vi "Post Media Tweet - From File.vi"(8 "error in":errorcluster, 9 "Picture File (PNG, JPG, GIF)":path, 10 "Tweet":string, 11 "Twitter Handle In":T1={"OAuth Credentials"={"Consumer Key"="", "Signature Method"=enum."HMAC-SHA1", "Token"="", "Version"="", "Token Secret"="", "Consumer Secret"=""}, "since ID"="", "max ID"="", "Screen Name"=""}) -> (0 "error out":errorcluster, 3 "Twitter Handle Out":T1={"OAuth Credentials"={"Consumer Key"="", "Signature Method"=enum."HMAC-SHA1", "Token"="", "Version"="", "Token Secret"="", "Consumer Secret"=""}, "since ID"="", "max ID"="", "Screen Name"=""})   [LabVIEW 2011, in "i3-twitter.lvlib"]
uses:
  i3-twitter.lvlib
  Controls/Twitter Handle.ctl
  i3-oauth/Controls/OAuth Credentials.ctl
  i3-oauth/Controls/Signature Method.ctl
  <vilib>/httpClient/MultipartData.ctl
  i3-oauth/Controls/HTTP Method.ctl
  i3-oauth/i3-oauth.lvlib
  <vilib>/httpClient/LabVIEWHTTPClient.lvlib
panel:
  out "headers (response)":string
  out "body (response)":string
  out "Full URL":string
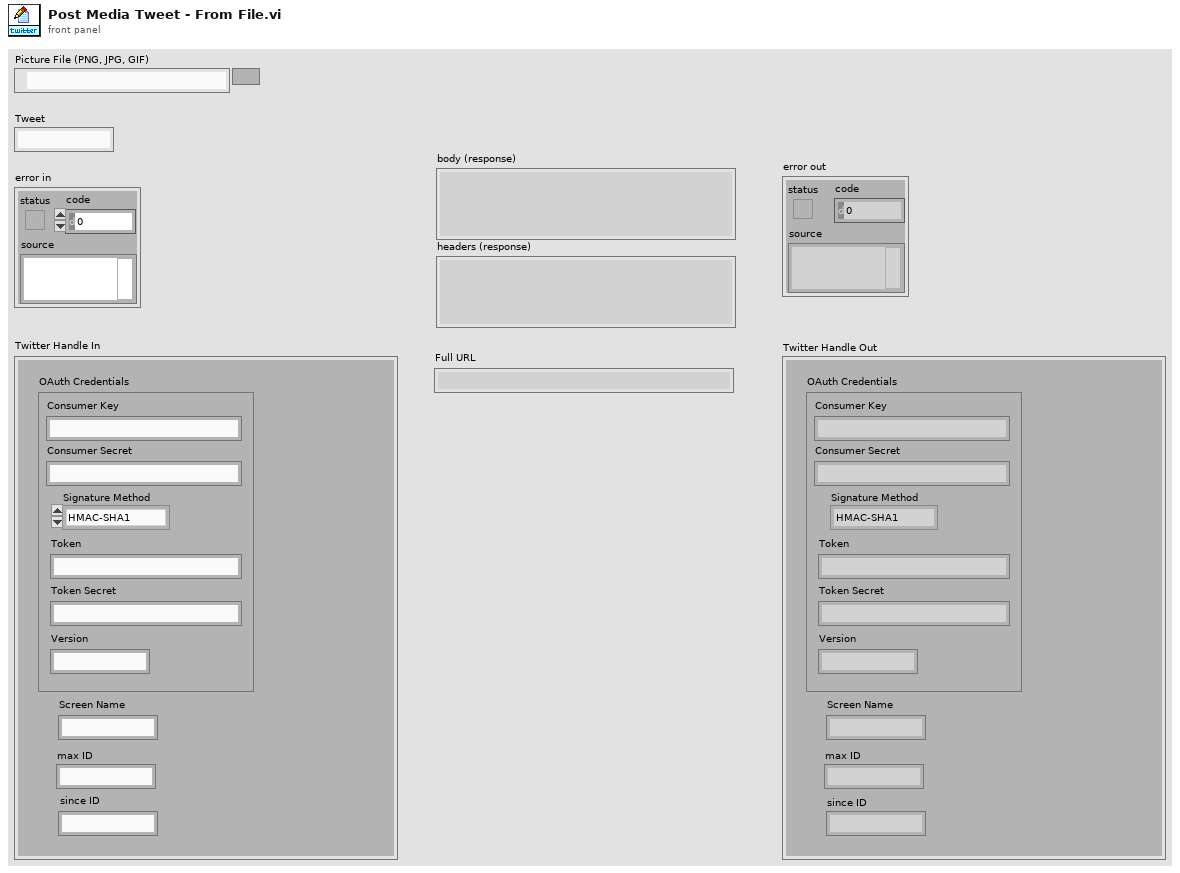
[diagram p1: front panel]
types:
  T1 = typedef "i3-twitter.lvlib/Twitter Handle.ctl" = cluster{"OAuth Credentials":T2, "since ID":string, "max ID":string, "Screen Name":string}
  T2 = typedef "i3-oauth.lvlib/OAuth Credentials.ctl" = cluster{"Consumer Key":string, "Signature Method":T3, "Token":string, "Version":string, "Token Secret":string, "Consumer Secret":string}
  T3 = typedef "i3-oauth.lvlib/Signature Method.ctl" = enum16{"HMAC-MD5", "HMAC-SHA1", "HMAC-SHA224", "HMAC-SHA256", "HMAC-SHA384", "HMAC-SHA512"}
  T4 = typedef "LabVIEWHTTPClient.lvlib/MultipartData.ctl" = cluster{"Name":string, "Value":string, "File":path, "Filename":string, "MIME type":string}
  T5 = typedef "i3-oauth.lvlib/HTTP Method.ctl" = enum16{"GET", "POST", "PUT", "DELETE"}
  T6 = typedef "LabVIEWHTTPClient.lvlib/ClientHandle.ctl" = refnum<k1>
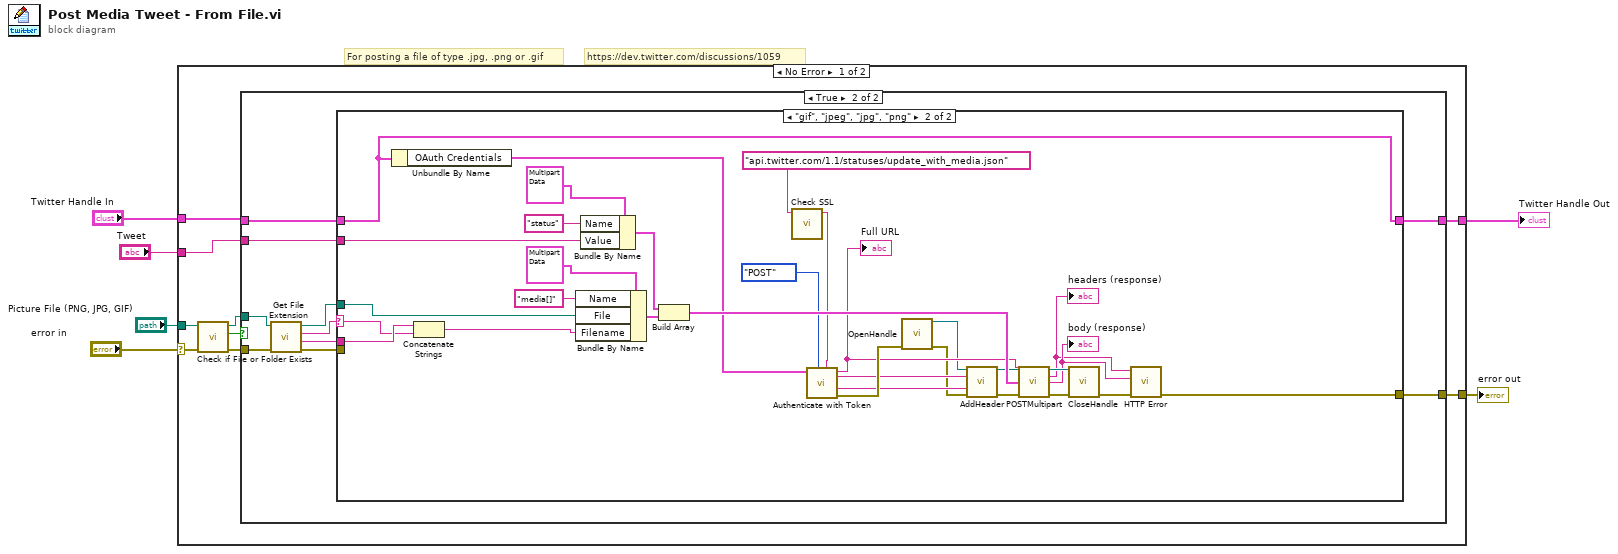
[diagram p0: block diagram]
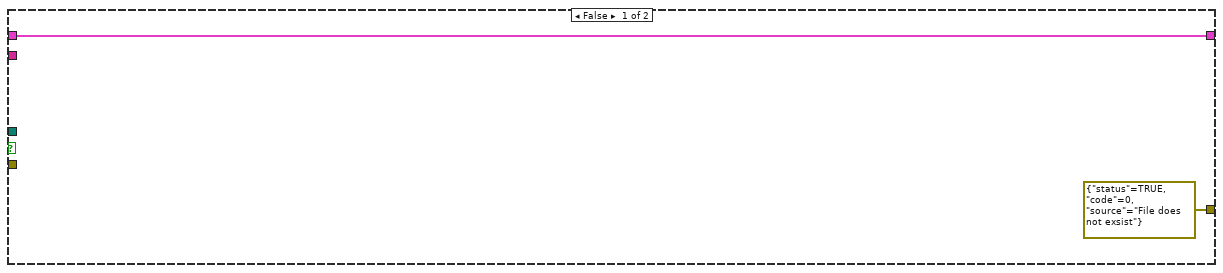
[diagram p2: hidden frame]
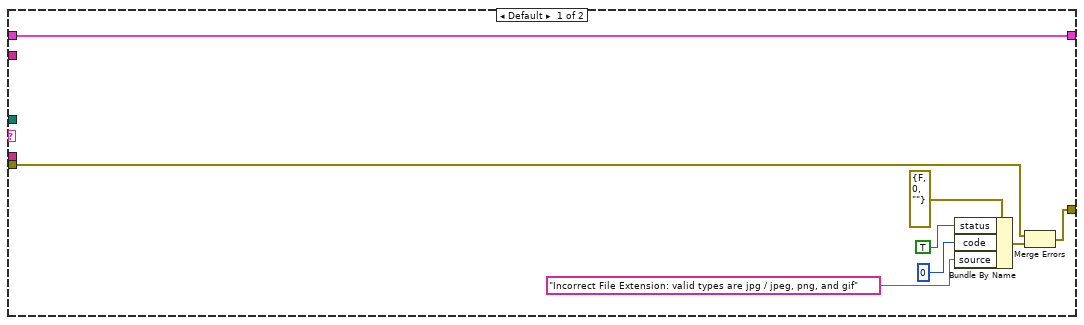
[diagram p3: hidden frame]
diagram:
  # "For posting a file of type .jpg, .png or .gif"
  # "https://dev.twitter.com/discussions/1059"
  n1 = case shown="No Error" "error in" {
    selector: "error in" -> [w7 w68]
    tunnel: [w15 w68] -> w5
    tunnel: "Picture File (PNG, JPG, GIF)" -> [w14 _]
    tunnel: "Twitter Handle In" -> [w11 w67]
    tunnel: "Tweet" -> [w10 _]
    tunnel: [w9 w67] -> w1
    frame No Error {
      n2 = call <vilib>:"Check if File or Folder Exists.vi"("error in (no error)"=w7, "path"=w14) -> ("error out"=w8:errorcluster, "file or folder exists?"=w13:bool, "dup path"=w12:path)  [unwired: 7 in]
      n3 = case shown="True" w13 {
        tunnel: [errorcluster {"status"=TRUE, "code"=0, "source"="File does not exsist"} ("error out") w27] -> w15
        tunnel: w12 -> [_ w26]
        tunnel: w11 -> [w16 w23]
        tunnel: w10 -> [_ w22]
        tunnel: [w16 w21] -> w9
        tunnel: w8 -> [_ w19]
        frame False {
        }
        frame True {
          n4 = call <vilib>:"Get File Extension.vi"("error in (no error)"=w19, "file"=w26) -> ("error out"=w18:errorcluster, "filename without extension"=w20:string, "lowercase file extension"=w25:string, "dup file"=w24:path)  [unwired: 6 in]
          n5 = case shown="\"gif\", \"jpeg\", \"jpg\", \"png\"" w25 {
            selector: w25 -> [_ w40]
            tunnel: [w29 w45] -> w27
            tunnel: w24 -> [_ w48]
            tunnel: w23 -> [w35 w42]
            tunnel: w22 -> [_ w47]
            tunnel: [w35 w42] -> w21
            tunnel: w20 -> [_ w41]
            tunnel: w18 -> [w28 _]
            frame Default {
              n6 = Bundle By Name(cluster=errorcluster {"status"=FALSE, "code"=0, "source"=""} ("error in (no error)"), "status"=TRUE, "code"=0, "source"="Incorrect File Extension: valid types are jpg / jpeg, png, and gif") -> (w30:errorcluster)
              n7 = Merge Errors(w28, w30) -> (w29:errorcluster)
            }
            frame "gif", "jpeg", "jpg", "png" {
              n8 = Unbundle By Name(w42) -> ("OAuth Credentials"=w38:T2)
              n9 = Concatenate Strings(w41, w40) -> (w49:string)
              n10 = Bundle By Name(cluster=T4 {"Name"="", "Value"="", "File"=path "", "Filename"="", "MIME type"="application/octet-stream"} ("Element"), "Name"="media[]", "File"=w48, "Filename"=w49) -> (w64:T4)
              n11 = Bundle By Name(cluster=T4 {"Name"="", "Value"="", "File"=path "", "Filename"="", "MIME type"="application/octet-stream"} ("Element"), "Name"="status", "Value"=w47) -> (w60:T4)
              n12 = Build Array(w60, w64) -> (w61:T4[])
              n13 = call "Check SSL.vi"("Input URL"="api.twitter.com/1.1/statuses/update_with_media.json" ("Base URL")) -> ("Output URL"=w37:string)  [unwired: 8 in]
              n14 = call "Authenticate with Token.vi"("Base URL"=w37, "HTTP Method"=HTTP_Method."POST", "OAuth Credentials"=w38) -> ("error out"=w66:errorcluster, "Header Value"=w53:string, "Header Parameter"=w52:string, "Full URL"=w58:string)  [unwired: 4 in, 1 out]
              "Full URL" <- w58
              n15 = call <vilib>:"OpenHandle.vi"("error in (no error)"=w66) -> ("client handle out"=w50:T6, "error out"=w51:errorcluster)  [unwired: 13 in]
              n16 = call <vilib>:"AddHeader.vi"("client handle"=w50, "header"=w52, "value"=w53, "error in (no error)"=w51) -> ("client handle out"=w54:T6, "error out"=w55:errorcluster)  [unwired: 10 in]
              n17 = call <vilib>:"POSTMultipart.vi"("client handle"=w54, "url"=w58, "data"=w61, "error in (no error)"=w55) -> ("client handle out"=w57:T6, "headers"=w43:string, "body"=w44:string, "error out"=w56:errorcluster)  [unwired: 8 in]
              "body (response)" <- w44
              "headers (response)" <- w43
              n18 = call <vilib>:"CloseHandle.vi"("client handle"=w57, "error in (no error)"=w56) -> ("error out"=w46:errorcluster)  [unwired: 13 in]
              n19 = call "HTTP Error.vi"("error in (no error)"=w46, "Body"=w44, "Header"=w43) -> ("error out"=w45:errorcluster)  [unwired: 6 in, 2 out]
            }
          }
        }
      }
    }
    frame Error {
    }
  }
  "error out" <- w5
  "Twitter Handle Out" <- w1
